vi "Fetch Measurement (Single Point).vi"(8 "error in (no error)":errorcluster, 9 "Data Mode (5: Voltage)":i32(ring)=5 items=["Current", "Resistance", "Source Output Setting", "Status", "Time", "Voltage"], 10 "Channel (0: Channel 1)":i32(ring) items=["Channel 1", "Channel 2"], 11 "VISA resource name":refnum<visa-resource-name>) -> (0 "error out":errorcluster, 2 "Measurement":dbl, 3 "VISA resource name out":refnum<visa-resource-name>)   [LabVIEW 2023, in "Agilent B2900 Series.lvlib"]
doc: "Returns the latest data of the voltage measurement, current measurement, resistance measurement, time, status, or source output setting.\n\n<B>Note:</B> Use this VI only with other low-level VIs. The high-level VIs automatically incorporate this functionality. This VI does not check the instrument status."
uses:
  Agilent B2900 Series.lvlib
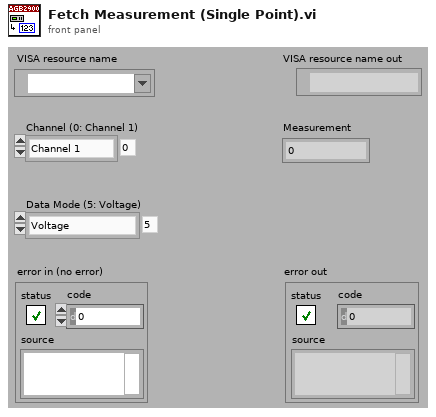
[diagram p1: front panel]
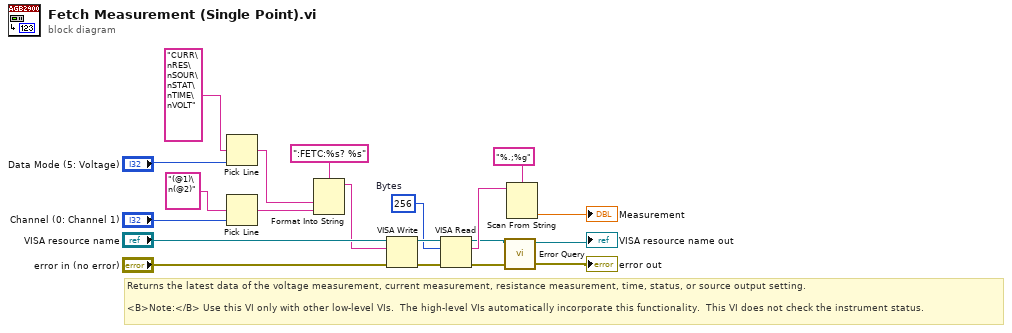
[diagram p0: block diagram]
diagram:
  w13 = u32 256  # Bytes
  # "Returns the latest data of the voltage measurement, current measurement, resistance measurement, time, status, or source output setting.\n\n<B>Note:</B> Use this VI only with other low-level VIs.  The high-level VIs automatically incorporate this functionality.  This VI does not check the instrument status."
  n1 = Pick Line(multi-line string="CURR\nRES\nSOUR\nSTAT\nTIME\nVOLT", line index="Data Mode (5: Voltage)") -> (output string=w16:string)  [unwired: 1 in]
  n2 = Pick Line(multi-line string="(@1)\n(@2)", line index="Channel (0: Channel 1)") -> (output string=w7:string)  [unwired: 1 in]
  n3 = Format Into String(format string=":FETC:%s? %s", w16, w7) -> (resulting string=w12:string)  [unwired: 2 in, 1 out]
  n4 = VISA Write(VISA resource name="VISA resource name", write buffer=w12, error in (no error)="error in (no error)") -> (VISA resource name out=w14:refnum<visa-resource-name>, error out=w15:errorcluster)  [unwired: 1 out]
  n5 = VISA Read(VISA resource name=w14, byte count=w13, error in (no error)=w15) -> (VISA resource name out=w4:refnum<visa-resource-name>, read buffer=w9:string, error out=w3:errorcluster)  [unwired: 1 out]
  n6 = call "Error Query.vi"("error in (no error)"=w3, "VISA resource name"=w4) -> ("error out"=→"error out":errorcluster, "VISA resource name out"=→"VISA resource name out":refnum<visa-resource-name>)  [unwired: 6 in, 2 out]
  n7 = Scan From String(format string="%.;%g", input string=w9) -> (output 1=→"Measurement":dbl)  [unwired: 3 in, 3 out]
